vi "External Interface.vi"() -> ()   [LabVIEW 2016]
uses:
  <vilib>/Plasmionique/MB Master/MB_Master_TCP/MB_Master_TCP.lvclass
  C:/Program Files (x86)/National Instruments/LabVIEW 2016/vi.lib/Plasmionique/MB Master/MB_Master/MB_Master.lvclass
  <vilib>/Plasmionique/MB Master/MB_Master/MB_Master.lvclass
  <vilib>/Plasmionique/MB Master/MB Master.lvlib
panel:
  in  "starting address 4":u16
  in  "values 4":u16[](array[numeric])
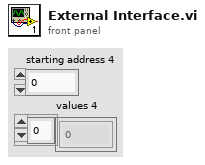
[diagram p1: front panel]
types:
  T1 = cluster{"COD浓度（mg/L)":dbl, "水样启动时间":timestamp, "加标回收启动时间":timestamp, "CODMn工作状态":enum16{"空闲", "水样测试", "标样核查", "零点核查", "跨度核查", "空白测试", "平行样测试", "加标回收", "空白校准", "标样校准", "初始化（清洗）"}, "多列列表框":i32}
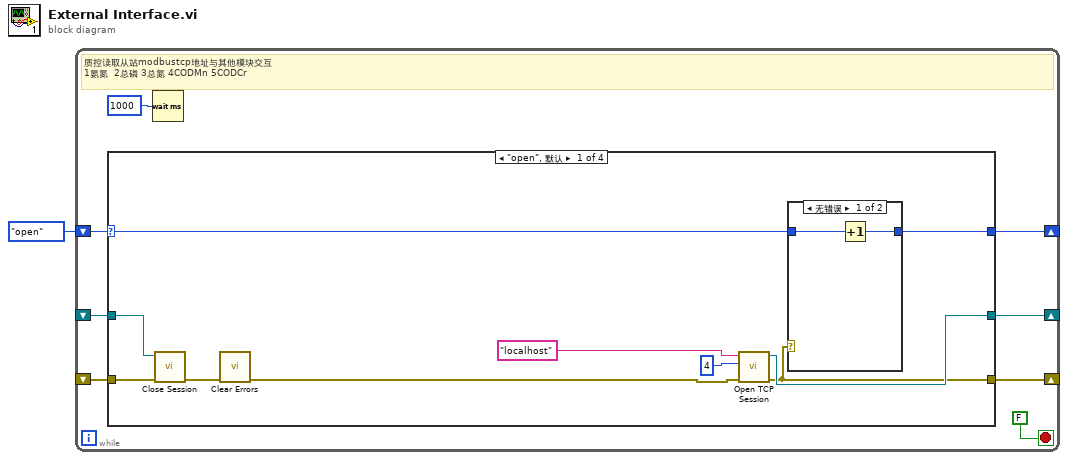
[diagram p0: block diagram]
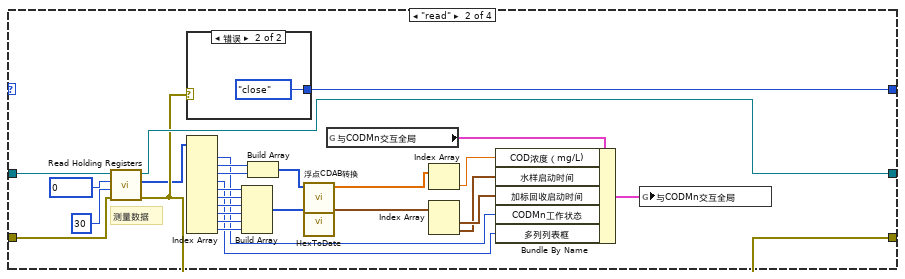
[diagram p3: hidden frame]
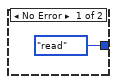
[diagram p4: hidden frame]
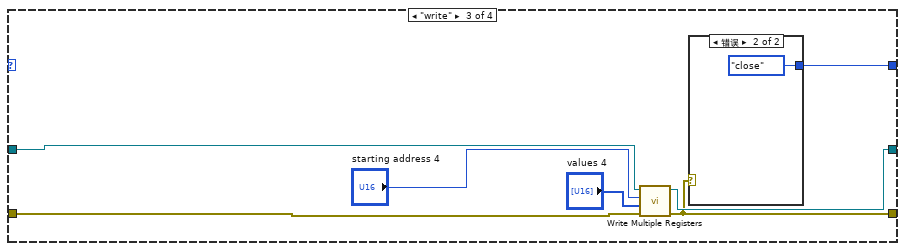
[diagram p5: hidden frame]
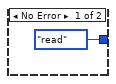
[diagram p6: hidden frame]
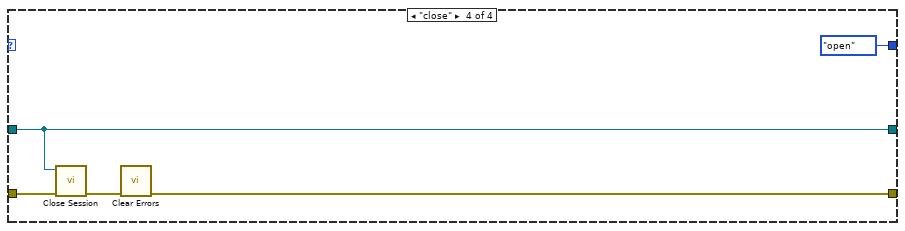
[diagram p7: hidden frame]
diagram:
  n1 = while {
    shift-right: [w7] -> _
    shift-left: _ -> [w9]
    shift-right: [w6] -> _
    shift-left: _ -> [w8]
    shift-right: [w3] -> _
    shift-left: enum16{"open", "read", "write", "close"}."open" -> [w4]
    stop <- FALSE stop-if-true
    # "质控读取从站modbustcp地址与其他模块交互\n1氨氮  2总磷 3总氮 4CODMn 5CODCr"
    n2 = case shown="\"open\", 默认" w4 {
      selector: w4 -> [w11 _ _ _]
      tunnel: w9 -> [w16 w49 w57 w65]
      tunnel: w8 -> [w15 w46 w56 w64]
      tunnel: [w17 w44 w55 w65] -> w7
      tunnel: [w12 w43 w54 w62] -> w6
      tunnel: [w10 w45 w58 enum16{"open", "read", "write", "close"}."open"] -> w3
      frame "open", Default {
        n3 = call-dynamic "Close Session.vi"("error in (no error)"=w15, "MB session in"=w16) -> ("error out"=w14:errorcluster)  [unwired: 9 in]
        n4 = call <vilib>:"Clear Errors.vi"("error in (no error)"=w14) -> ("error out"=w13:errorcluster)  [unwired: 5 in, 1 out]
        n5 = call <vilib>:"Open TCP Session.vi"("error in (no error)"=w13, "Port (502)"=u16 4, "IP Address"="localhost") -> ("error out"=w12:errorcluster, "MB_TCP session"=w17:refnum<class "MB_Master_TCP.lvclass">)  [unwired: 7 in]
        n6 = case shown="无错误" w12 {
          tunnel: w11 -> [w21 w22]
          tunnel: [w20 w22] -> w10
          frame No Error {
            n7 = Increment(x=w21) -> (x+1=w20:enum16{"open", "read", "write", "close"})
          }
          frame Error {
          }
        }
      }
      frame "read" {
        # "测量数据"
        n8 = call <vilib>:"Read Holding Registers.vi"("error in (no error)"=w46, "quantity"=u16 30, "starting address"=u16 0, "MB session in"=w49) -> ("error out"=w43:errorcluster, "Registers"=w42:u16[], "MB session out"=w44:refnum<class "MB_Master.lvclass">)  [unwired: 5 in]
        n9 = case shown="错误" w43 {
          tunnel: [enum16{"open", "read", "write", "close"}."read" enum16{"open", "read", "write", "close"}."close"] -> w45
          frame No Error {
          }
          frame Error {
          }
        }
        n10 = Index Array(array=w42) -> (element #1=w26:u16, element #2=w41:u16, element #3=w40:u16, element #4=w25:u16, element #5=w37:u16, element #6=w36:u16, element #7=w35:u16, element #8=w33:u16, element #9=w32:u16, element #10=w31:u16)  [unwired: 10 in]
        n11 = Build Array(w37, w36, w35, w33, w32, w31) -> (w34:u16[])
        n12 = Build Array(w41, w40) -> (w39:u16[])
        n13 = call "浮点CDAB转换.vi"("数组"=w39) -> ("数组 2"=w38:sgl[])  [unwired: 10 in]
        n14 = call "HexToDate.vi"("数组"=w34) -> ("DATE"=w30:timestamp[])  [unwired: 10 in]
        n15 = global read "modbus slave全局.vi" "与CODMn交互全局"() -> (w28:T1)
        n16 = Index Array(array=w38) -> (element=w27:sgl)  [unwired: 1 in]
        n17 = Index Array(array=w30) -> (element #1=w24:timestamp, element #2=w23:timestamp)  [unwired: 2 in]
        n18 = Bundle By Name(cluster=w28, "COD浓度（mg/L)"=w27, "水样启动时间"=w23, "加标回收启动时间"=w24, "CODMn工作状态"=w26, "多列列表框"=w25) -> (w29:T1)
        n19 = global write "modbus slave全局.vi" "与CODMn交互全局"(w29) -> ()
      }
      frame "write" {
        n20 = call <vilib>:"Write Multiple Registers.vi"("error in (no error)"=w56, "values"="values 4", "starting address"="starting address 4", "MB session in"=w57) -> ("error out"=w54:errorcluster, "MB session out"=w55:refnum<class "MB_Master.lvclass">)  [unwired: 6 in]
        n21 = case shown="错误" w54 {
          tunnel: [enum16{"open", "read", "write", "close"}."read" enum16{"open", "read", "write", "close"}."close"] -> w58
          frame No Error {
          }
          frame Error {
          }
        }
      }
      frame "close" {
        n22 = call-dynamic "Close Session.vi"("error in (no error)"=w64, "MB session in"=w65) -> ("error out"=w63:errorcluster)  [unwired: 9 in]
        n23 = call <vilib>:"Clear Errors.vi"("error in (no error)"=w63) -> ("error out"=w62:errorcluster)  [unwired: 5 in, 1 out]
      }
    }
    n24 = Wait (ms)(milliseconds to wait=u32 1000 ("等待时间（毫秒）")) -> ()  [unwired: 1 out]
  }
